vi "DataType_Init.vi"(0 "object in":refnum<class "DataType.lvclass">, 2 "Data Method":refnum<class "IDataMethod.lvclass">, 5 "error in (no error)":errorcluster) -> (14 "object out":refnum<class "DataType.lvclass">, 19 "error out":errorcluster)   [LabVIEW 2024, in "DataType.lvclass"]
uses:
  DataType.lvclass
  DataType.lvclass/DataType.ctl
  IDataMethod_interface/IDataMethod.lvclass
panel:
  # "Connector Pane"
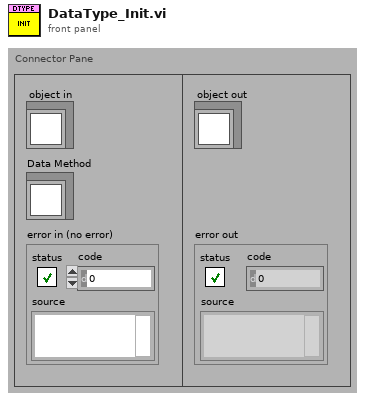
[diagram p1: front panel]
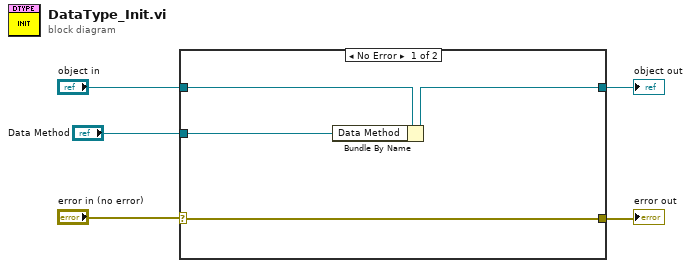
[diagram p0: block diagram]
diagram:
  n1 = case shown="No Error" "error in (no error)" {
    selector: "error in (no error)" -> [w7 w10]
    tunnel: "object in" -> [w9 w11]
    tunnel: [w8 w11] -> w4
    tunnel: [w7 w10] -> w2
    tunnel: "Data Method" -> [w6 _]
    frame No Error {
      n2 = Bundle By Name(cluster=w9, "Data Method"=w6) -> (w8:refnum<class "DataType.lvclass">)
    }
    frame Error {
    }
  }
  "object out" <- w4
  "error out" <- w2
